vi "Update Modifying When Mouse Up.vi"(8 "error in (no error)":errorcluster, 11 "Canvas in":refnum<class "Canvas.lvclass">) -> (0 "error out":errorcluster, 3 "Canvas out":refnum<class "Canvas.lvclass">)   [LabVIEW 2015, in "Canvas.lvclass"]
uses:
  Canvas.lvclass
  Canvas.lvclass/Canvas.ctl
  Graphic/Graphic.lvclass/Graphic.ctl
  Scalable Border/Scalable Border.lvclass
  Graphic/Graphic.lvclass
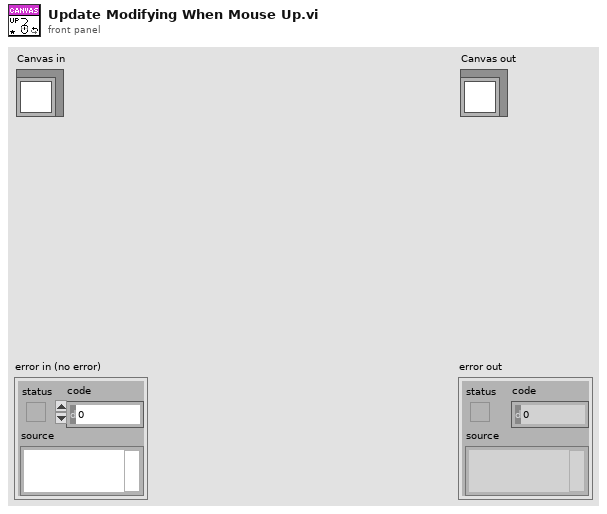
[diagram p1: front panel]
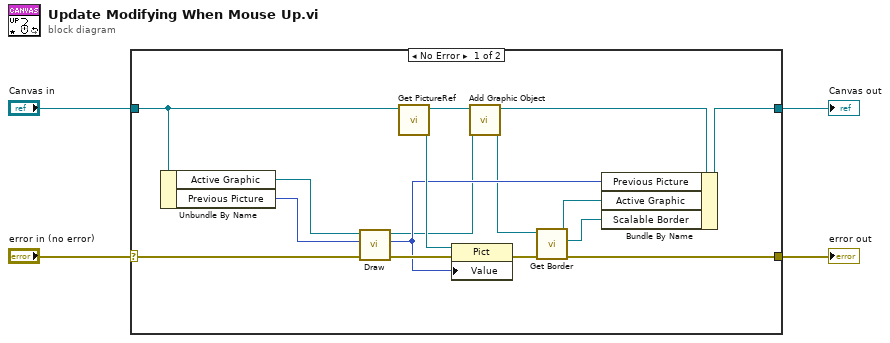
[diagram p0: block diagram]
diagram:
  n1 = case shown="No Error" "error in (no error)" {
    selector: "error in (no error)" -> [w18 w22]
    tunnel: [w10 w22] -> w3
    tunnel: [w20 w21] -> w1
    tunnel: "Canvas in" -> [w19 w21]
    frame No Error {
      n2 = Unbundle By Name(w19) -> ("Active Graphic"=w11:refnum<class "Graphic.lvclass">, "Previous Picture"=w6:picture)
      n3 = call-dynamic "Draw.vi"("error in (no error)"=w18, "Picture in"=w6, "Graphic in"=w11) -> ("error out"=w15:errorcluster, "Picture out"=w12:picture, "Graphic out"=w9:refnum<class "Graphic.lvclass">)  [unwired: 6 in]
      n4 = call "Get PictureRef.vi"("Canvas in"=w19) -> ("PictureRef"=w14:refnum<vi>, "Canvas out"=w16:refnum<class "Canvas.lvclass">)  [unwired: 8 in, 1 out]
      n5 = property class="Pict"(reference=w14, error in=w15, "Value"=w12) -> (error out=w17:errorcluster)  [unwired: 1 out]
      n6 = call "Add Graphic Object.vi"("Graphic"=w9, "Canvas in"=w16) -> ("Graphic out"=w5:refnum<class "Graphic.lvclass">, "Canvas out"=w13:refnum<class "Canvas.lvclass">)  [unwired: 7 in, 1 out]
      n7 = call "Get Border.vi"("error in (no error)"=w17, "Graphic in"=w5) -> ("error out"=w10:errorcluster, "Scalable Border.lvclass"=w7:refnum<class "Scalable Border.lvclass">, "Graphic out"=w8:refnum<class "Graphic.lvclass">)  [unwired: 7 in]
      n8 = Bundle By Name(cluster=w13, "Previous Picture"=w12, "Active Graphic"=w8, "Scalable Border"=w7) -> (w20:refnum<class "Canvas.lvclass">)
    }
    frame Error {
    }
  }
  "error out" <- w3
  "Canvas out" <- w1
